vi "AbsoluteMove.vi"(0 "CmdLib In":refnum<k24>, 1 "DeviceKey In":string, 2 "Device Address In":i32, 3 "Motor":i32, 4 "Target Pos":i32, 5 "error in (no error)":errorcluster, 6 "执行":bool) -> (14 "CmdLib Out":refnum<k24>, 16 "DeviceKey Out":string, 17 "Device Address Out":i32, 19 "error out":errorcluster)   [LabVIEW 2018]
uses:
  Device VIs/CmdLib.dll
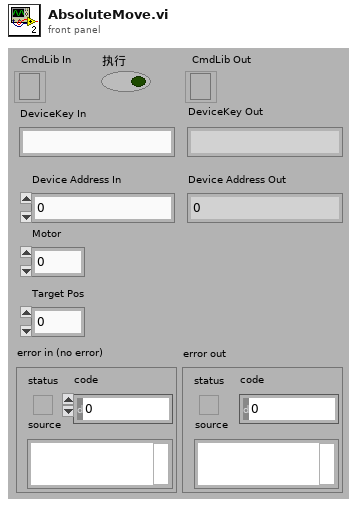
[diagram p1: front panel]
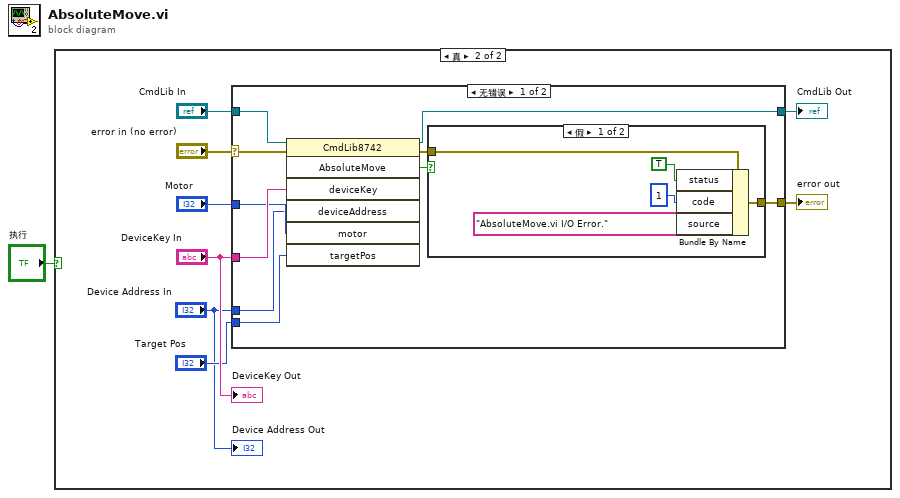
[diagram p0: block diagram]
diagram:
  n1 = case shown="真" "执行" {
    frame False {
    }
    frame True {
      n2 = case shown="无错误" "error in (no error)" {
        selector: "error in (no error)" -> [w16 w26]
        tunnel: "CmdLib In" -> [w19 w27]
        tunnel: [w18 w27] -> w8
        tunnel: "Motor" -> [w11 _]
        tunnel: "DeviceKey In" -> [w17 _]
        tunnel: [w13 w26] -> w5
        tunnel: "Target Pos" -> [w12 _]
        tunnel: "Device Address In" -> [w10 _]
        frame No Error {
          n3 = invoke class="CmdLib8742" method="AbsoluteMove"(reference=w19, error in=w16, "deviceKey"=w17, "deviceAddress"=w10, "motor"=w11, "targetPos"=w12) -> (reference out=w18:refnum<k24>, error out=w14:errorcluster, "AbsoluteMove"=w15:bool)  [unwired: 1 in, 4 out]
          n4 = case shown="假" w15 {
            tunnel: w14 -> [w24 w25]
            tunnel: [w23 w25] -> w13
            frame False {
              n5 = Bundle By Name(cluster=w24, "status"=TRUE, "code"=1, "source"="AbsoluteMove.vi I/O Error.") -> (w23:errorcluster)
            }
            frame True {
            }
          }
        }
        frame Error {
        }
      }
      "error out" <- w5
      "CmdLib Out" <- w8
      "DeviceKey Out" <- "DeviceKey In"
      "Device Address Out" <- "Device Address In"
    }
  }
